vi "addParameterURL.vi"(9 "Parameter Value":string="ok", 10 "Parameter Key":string="test", 11 "Command URL in":string) -> (2 "Command URL out":string)   [LabVIEW 2019, in "PF_API.lvclass"]
uses:
  PF_API.lvclass
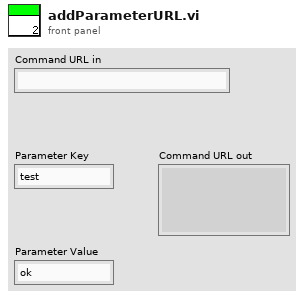
[diagram p1: front panel]
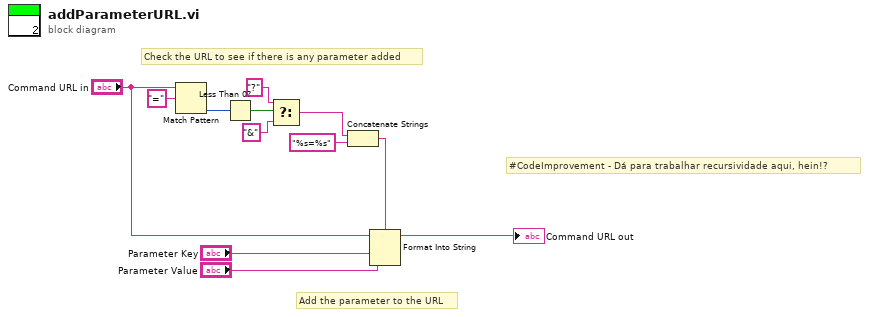
[diagram p0: block diagram]
diagram:
  # "#CodeImprovement - Dá para trabalhar recursividade aqui, hein!?"
  # "Add the parameter to the URL"
  # "Check the URL to see if there is any parameter added"
  n1 = Match Pattern(string="Command URL in", regular expression="=") -> (offset past match=w6:i32)  [unwired: 1 in, 3 out]
  n2 = Less Than 0?(x=w6) -> (x < 0?=w5:bool)
  n3 = Select(t="?" ("regular expression"), s=w5, f="&" ("regular expression")) -> (s? t:f=w2:string)
  n4 = Concatenate Strings(w2, "%s=%s" ("format string")) -> (w8:string)
  n5 = Format Into String(format string=w8, initial string="Command URL in", "Parameter Key", "Parameter Value") -> (resulting string=→"Command URL out":string)  [unwired: 1 in, 1 out]
